vi "8 Bit to 64 Bit (SubVI).vi"(8 "Input Valid":bool, 11 "Pixel Data (8-Bit)":u8) -> (0 "Output Valid":bool, 3 "Pixel Data (64-Bit)":u64)   [LabVIEW 2014]
uses:
  8 Bit to 64 Bit.ctl
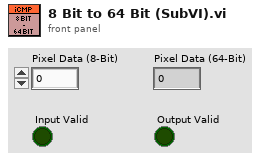
[diagram p1: front panel]
types:
  T1 = typedef "8 Bit to 64 Bit.ctl" = enum16{"Bit 0", "1", "2", "3", "4", "5", "6", "7"}
  T2 = cluster{"initialized array[0]":u8, "initialized array[1]":u8, "initialized array[2]":u8, "initialized array[3]":u8, "initialized array[4]":u8, "initialized array[5]":u8, "initialized array[6]":u8, "initialized array[7]":u8}
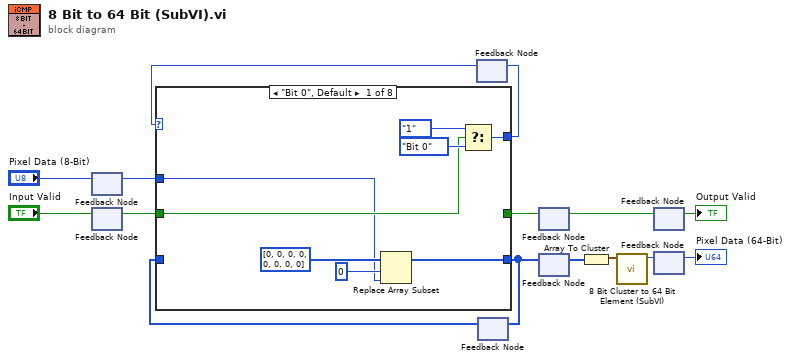
[diagram p0: block diagram]
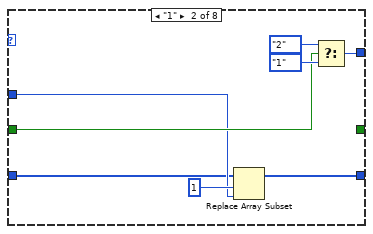
[diagram p2: hidden frame]
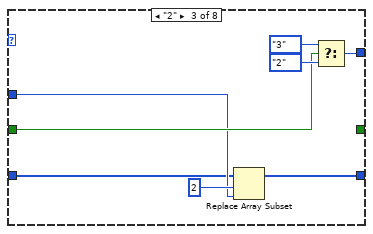
[diagram p3: hidden frame]
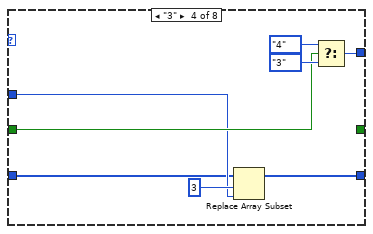
[diagram p4: hidden frame]
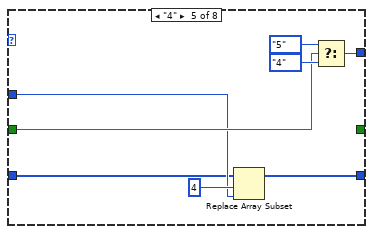
[diagram p5: hidden frame]
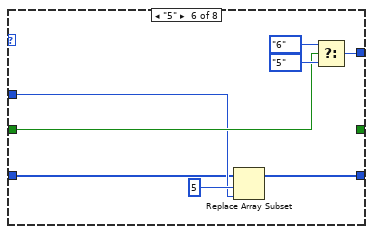
[diagram p6: hidden frame]
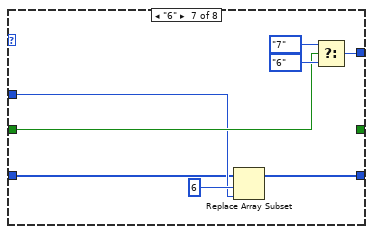
[diagram p7: hidden frame]
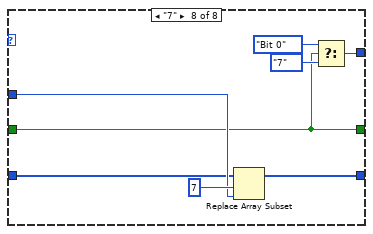
[diagram p8: hidden frame]
diagram:
  n1 = feedback-in #1("Pixel Data (8-Bit)") -> ()
  n2 = feedback #1() -> (w6:u8)  [unwired: 1 in]
  n3 = feedback-in #2("Input Valid") -> ()
  n4 = feedback #2() -> (w5:bool)  [unwired: 1 in]
  n5 = feedback #3() -> (w9:T1)  [unwired: 1 in]
  n6 = feedback #4() -> (w11:u8[])  [unwired: 1 in]
  n7 = case shown="\"Bit 0\", Default" w9 {
    tunnel: w5 -> [w21 w29 w37 w45 w53 w61 w69 w72]
    tunnel: [w20 w28 w36 w44 w52 w60 w68 w77] -> w8
    tunnel: w6 -> [w17 w26 w34 w42 w50 w58 w66 w75]
    tunnel: [w16 w25 w33 w41 w49 w57 w65 w74] -> w12
    tunnel: w11 -> [_ w24 w32 w40 w48 w56 w64 w73]
    tunnel: [_ _ _ _ _ _ _ w72] -> w15
    frame "Bit 0", Default {
      n8 = Replace Array Subset(array=u8[] [0, 0, 0, 0, 0, 0, 0, 0] ("initialized array"), new element=w17, index=0) -> (w16:u8[])
      n9 = Select(t=8_Bit_to_64_Bit."1", s=w21, f=8_Bit_to_64_Bit."Bit 0") -> (s? t:f=w20:T1)
    }
    frame "1" {
      n10 = Replace Array Subset(array=w24, new element=w26, index=1) -> (w25:u8[])
      n11 = Select(t=8_Bit_to_64_Bit."2", s=w29, f=8_Bit_to_64_Bit."1") -> (s? t:f=w28:T1)
    }
    frame "2" {
      n12 = Replace Array Subset(array=w32, new element=w34, index=2) -> (w33:u8[])
      n13 = Select(t=8_Bit_to_64_Bit."3", s=w37, f=8_Bit_to_64_Bit."2") -> (s? t:f=w36:T1)
    }
    frame "3" {
      n14 = Replace Array Subset(array=w40, new element=w42, index=3) -> (w41:u8[])
      n15 = Select(t=8_Bit_to_64_Bit."4", s=w45, f=8_Bit_to_64_Bit."3") -> (s? t:f=w44:T1)
    }
    frame "4" {
      n16 = Replace Array Subset(array=w48, new element=w50, index=4) -> (w49:u8[])
      n17 = Select(t=8_Bit_to_64_Bit."5", s=w53, f=8_Bit_to_64_Bit."4") -> (s? t:f=w52:T1)
    }
    frame "5" {
      n18 = Replace Array Subset(array=w56, new element=w58, index=5) -> (w57:u8[])
      n19 = Select(t=8_Bit_to_64_Bit."6", s=w61, f=8_Bit_to_64_Bit."5") -> (s? t:f=w60:T1)
    }
    frame "6" {
      n20 = Replace Array Subset(array=w64, new element=w66, index=6) -> (w65:u8[])
      n21 = Select(t=8_Bit_to_64_Bit."7", s=w69, f=8_Bit_to_64_Bit."6") -> (s? t:f=w68:T1)
    }
    frame "7" {
      n22 = Replace Array Subset(array=w73, new element=w75, index=7) -> (w74:u8[])
      n23 = Select(t=8_Bit_to_64_Bit."Bit 0", s=w72, f=8_Bit_to_64_Bit."7") -> (s? t:f=w77:T1)
    }
  }
  n24 = feedback-in #3(w8) -> ()
  n25 = feedback-in #4(w12) -> ()
  n26 = feedback-in #5(w15) -> ()
  n27 = feedback #5() -> (w2:bool)  [unwired: 1 in]
  n28 = feedback-in #6(w12) -> ()
  n29 = feedback #6() -> (w1:u8[])  [unwired: 1 in]
  n30 = Array To Cluster(array=w1) -> (cluster=w13:T2)
  n31 = call "8 Bit Cluster to 64 Bit Element (SubVI).vi"("Pixel Cluster"=w13) -> ("Pixel Data (64-Bit)"=w14:u64)  [unwired: 10 in]
  n32 = feedback-in #7(w2) -> ()
  n33 = feedback #7() -> (→"Output Valid":bool)  [unwired: 1 in]
  n34 = feedback-in #8(w14) -> ()
  n35 = feedback #8() -> (→"Pixel Data (64-Bit)":u64)  [unwired: 1 in]
